vi "Main.vi"() -> ()   [LabVIEW 2010, in "Labricks.lvlib"]
doc: "This is the main VI of the Labricks game."
uses:
  Labricks.lvlib
  <vilib>/Utility/miscctls.llb/LVPoint32TypeDef.ctl
  Game_class/Game.lvclass
panel:
  out "3D Picture":refnum<vi>(3d-picture)
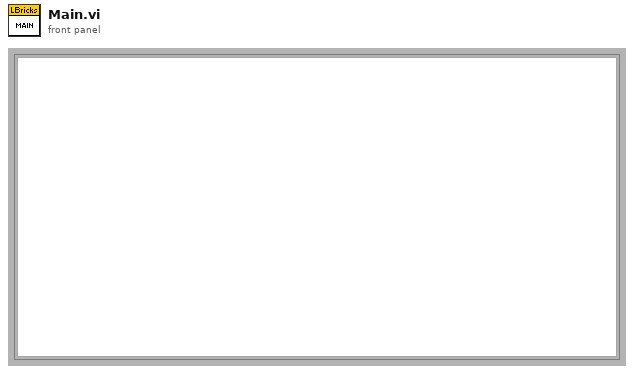
[diagram p1: front panel]
types:
  T1 = typedef "LVPoint32TypeDef.ctl" = cluster{"Horizontal":i32, "Vertical":i32}
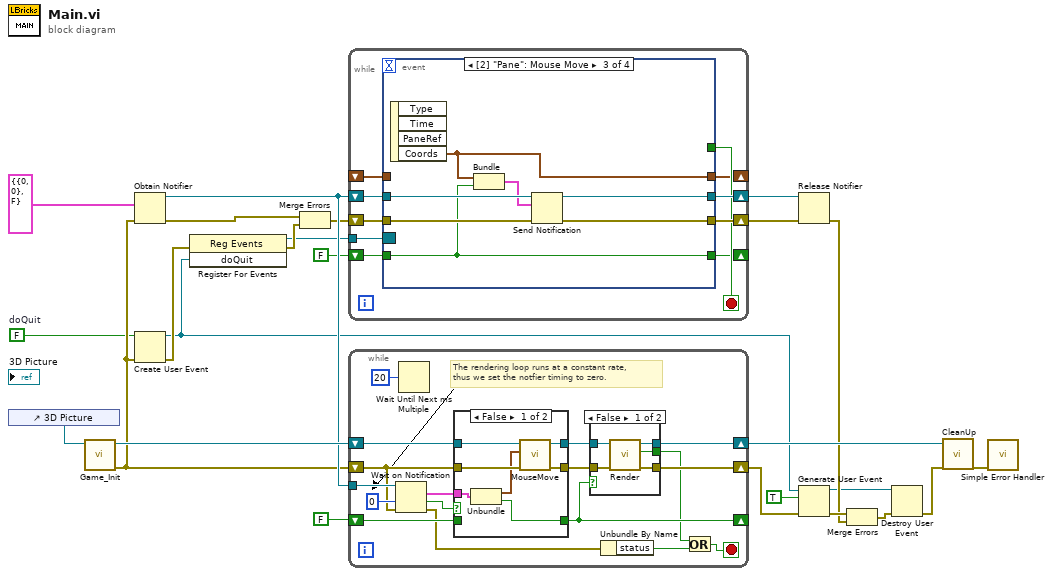
[diagram p0: block diagram]
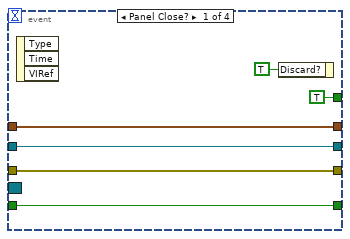
[diagram p2: hidden frame]
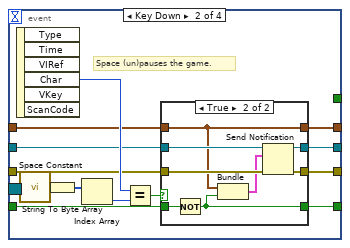
[diagram p3: hidden frame]
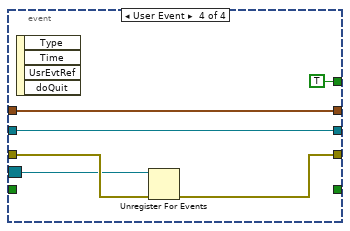
[diagram p5: hidden frame]
diagram:
  w17 = FALSE  # doQuit
  n1 = control-ref of="3D Picture"() -> (w11:refnum<vi>)
  n2 = call "Game_Init.vi"("display in"=w11) -> ("error out"=w18:errorcluster, "class data out"=w25:refnum<class "Game.lvclass">)  [unwired: 9 in]
  n3 = Obtain Notifier(notification data type=cluster{"coords in":T1, bool} {"coords in"={"Horizontal"=0, "Vertical"=0}, FALSE}, error in (no error)=w18) -> (notifier out=w21:refnum<notifier>, error out=w15:errorcluster)  [unwired: 2 in, 1 out]
  n4 = Create User Event(user event datatype=w17, error in=w18) -> (user event=w4:refnum<user-event>, error out=w14:errorcluster)
  n5 = register-events(error in=w14, w4) -> (reference out=w12:refnum<event-registration>, error out=w13:errorcluster)  [unwired: 1 in]
  n6 = Merge Errors(w15, w13) -> (w16:errorcluster)
  n7 = while {
    shift-right: [w34] -> w20
    shift-left: w21 -> [w35]
    shift-right: [w32] -> w10
    shift-left: w16 -> [w33]
    shift-right: [w29] -> _
    shift-left: FALSE -> [w30]
    tunnel: w12 -> [w28]
    shift-right: [w27] -> _
    shift-left: _ -> [w26]
    stop <- w31 stop-if-true
    n8 = event shown="[2] \"Pane\": Mouse Move" {
      selector: w28 -> [_ _ _ w75]
      dyn-events: _ -> [_ _ _ _]
      timeout: _ -> [_ _ _ _]
      tunnel: [TRUE ("quit out") _ _ TRUE ("quit out")] -> w31
      tunnel: w35 -> [w41 w45 w70 w79]
      tunnel: [w41 w44 w71 w79] -> w34
      tunnel: w33 -> [w40 w43 w73 w77]
      tunnel: [w40 w42 w72 w76] -> w32
      tunnel: w30 -> [w37 w52 w68 _]
      tunnel: [w37 w53 w68 _] -> w29
      tunnel: [w36 w47 w67 w74] -> w27
      tunnel: w26 -> [w36 w46 _ w74]
      event Panel Close? {
        n9 = event-data() -> ()  [unwired: 1 in, 3 out]
        n10 = event-data("Discard?"=TRUE) -> ()  [unwired: 1 in, 1 out]
      }
      event Key Down {
        # "Space (un)pauses the game."
        n11 = event-data() -> ("Char"=w51:i16)  [unwired: 1 in, 5 out]
        n12 = call <vilib>:"Space Constant.vi"() -> ("String"=w50:string)
        n13 = String To Byte Array(string=w50) -> (unsigned byte array=w49:u8[])
        n14 = Index Array(array=w49) -> (element=w48:u8)  [unwired: 1 in]
        n15 = Equal?(x=w51, y=w48) -> (x = y?=w54:bool)
        n16 = case shown="True" w54 {
          tunnel: [w58 w60] -> w53
          tunnel: w52 -> [w58 w66]
          tunnel: [w57 w61] -> w47
          tunnel: w46 -> [w57 w61]
          tunnel: w45 -> [w56 w65]
          tunnel: [w56 w64] -> w44
          tunnel: w43 -> [w55 w63]
          tunnel: [w55 w62] -> w42
          frame False {
          }
          frame True {
            n17 = Not(x=w66) -> (.not. x?=w60:bool)
            n18 = Bundle("Coords"=w61, w60) -> (w59:cluster{"Coords":T1, bool})  [unwired: 1 in]
            n19 = Send Notification(notification=w59, notifier=w65, error in (no error)=w63) -> (notifier out=w64:refnum<notifier>, error out=w62:errorcluster)
          }
        }
      }
      event Mouse Move {
        n20 = event-data() -> ("Coords"=w67:T1)  [unwired: 1 in, 3 out]
        n21 = Bundle("Coords"=w67, w68) -> (w69:cluster{"Coords":T1, bool})  [unwired: 1 in]
        n22 = Send Notification(notification=w69, notifier=w70, error in (no error)=w73) -> (notifier out=w71:refnum<notifier>, error out=w72:errorcluster)
      }
      event User Event {
        n23 = event-data() -> ()  [unwired: 1 in, 4 out]
        n24 = Unregister For Events(event registration refnum=w75, error in=w77) -> (error out=w76:errorcluster)
      }
    }
  }
  n25 = while {
    shift-right: [w93] -> w23
    shift-left: w25 -> [w96]
    shift-right: [w85] -> w9
    shift-left: w18 -> [w82]
    shift-right: [w87] -> _
    shift-left: FALSE -> [w88]
    tunnel: w21 -> [w90]
    stop <- w86 stop-if-true
    # "The rendering loop runs at a constant rate,\nthus we set the notfier timing to zero."
    n26 = Wait on Notification(notifier=w90, timeout in ms (-1)=0, error in (no error)=w82) -> (notification=w89:cluster{"coords in":T1, bool}, timed out?=w91:bool, error out=w83:errorcluster)  [unwired: 1 in, 1 out]
    n27 = Wait Until Next ms Multiple(millisecond multiple=u32 20) -> ()  [unwired: 1 out]
    n28 = case shown="False" w91 {
      tunnel: w96 -> [w103 w104]
      tunnel: [w102 w104] -> w95
      tunnel: [w101 w105] -> w94
      tunnel: w82 -> [w100 w105]
      tunnel: w89 -> [w99 _]
      tunnel: w88 -> [_ w106]
      tunnel: [w97 w106] -> w87
      frame False {
        n29 = Unbundle(w99) -> ("coords in"=w98:T1, w97:bool)
        n30 = call "MouseMove.vi"("error in"=w100, "coords in"=w98, "class data in"=w103) -> ("error out"=w101:errorcluster, "class data out"=w102:refnum<class "Game.lvclass">)  [unwired: 7 in]
      }
      frame True {
      }
    }
    n31 = case shown="False" w87 {
      tunnel: [w111 w113] -> w93
      tunnel: [w110 _] -> w81
      tunnel: w94 -> [w109 w112]
      tunnel: [w108 w112] -> w85
      tunnel: w95 -> [w107 w113]
      frame False {
        n32 = call "Render.vi"("error in"=w109, "class data in"=w107) -> ("error out"=w108:errorcluster, "quit out"=w110:bool, "class data out"=w111:refnum<class "Game.lvclass">)  [unwired: 7 in]
      }
      frame True {
      }
    }
    n33 = Unbundle By Name(w83) -> ("status"=w84:bool)
    n34 = Or(x=w81, y=w84) -> (x .or. y?=w86:bool)
  }
  n35 = Release Notifier(notifier=w20, error in (no error)=w10) -> (error out=w6:errorcluster)  [unwired: 1 in, 2 out]
  n36 = Generate User Event(user event=w4, event data cluster=TRUE ("event data"), error in=w9) -> (user event out=w3:refnum<user-event>, error out=w7:errorcluster)
  n37 = Merge Errors(w7, w6) -> (w5:errorcluster)
  n38 = Destroy User Event(user event=w3, error in=w5) -> (error out=w2:errorcluster)
  n39 = call-dynamic "CleanUp.vi"("class data in"=w23, "error in"=w2) -> ("error out"=w1:errorcluster)  [unwired: 16 in, 1 out]
  n40 = call <vilib>:"Simple Error Handler.vi"("error in (no error)"=w1) -> ()  [unwired: 4 in, 5 out]
